vi "RestartImagingWNewParameters.vi"(8 "error IO":errorcluster, 11 "notifier out":refnum<notifier>) -> (0 "error out 2":errorcluster)   [LabVIEW 2015]
uses:
  NIDAQControls/StateGlobals.vi
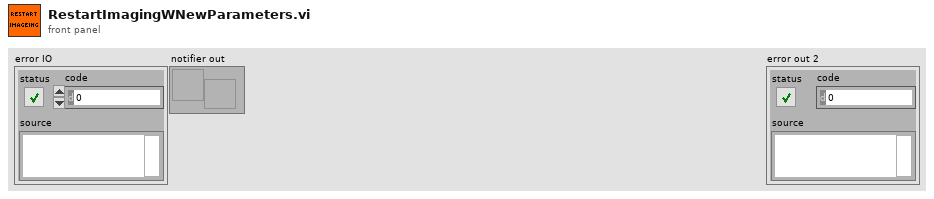
[diagram p1: front panel]
types:
  T1 = enum16{"Create", "Lossy Enqueue", "Enqueue", "Dequeue", "Destroy"}
  T2 = enum32{"Invalid", "Standard", "Closed", "Hidden", "Minimized", "Maximized"}
  T3 = cluster{"Start or New Parameters?":bool, "Laser Mode":string, "Piezo Mode":string, "Begin Or End Acquisition":string, "Acquisition Time":dbl}
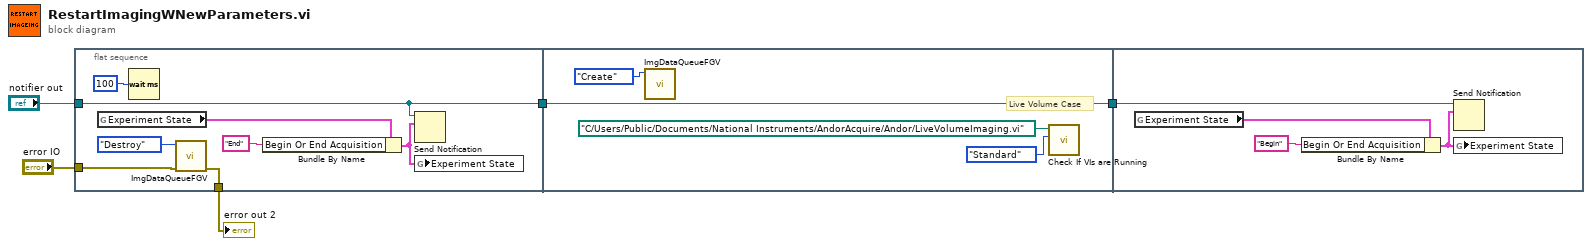
[diagram p0: block diagram]
diagram:
  n1 = flat-sequence {
    tunnel: "notifier out" -> [w6]
    tunnel: [w6] -> w5
    tunnel: "error IO" -> [w8]
    tunnel: [w7] -> w2
    tunnel: w5 -> [w17]
    tunnel: [w17] -> w4
    tunnel: w4 -> [w21]
    frame #0 {
      n2 = global read "StateGlobals.vi" "Experiment State"() -> (w13:T3)
      n3 = Wait (ms)(milliseconds to wait=u32 100) -> ()  [unwired: 1 out]
      n4 = call "ImgDataQueueFGV.vi"("error out"=w8, "Action"=T1."Destroy") -> ("error out 2"=w7:errorcluster)  [unwired: 7 in, 2 out]
      n5 = Bundle By Name(cluster=w13, "Begin Or End Acquisition"="End") -> (w11:T3)
      n6 = Send Notification(notification=w11, notifier=w6) -> ()  [unwired: 1 in, 2 out]
      n7 = global write "StateGlobals.vi" "Experiment State"(w11) -> ()
    }
    frame #1 {
      # "Live Volume Case"
      n8 = call "ImgDataQueueFGV.vi"("Action"=T1."Create") -> ()  [unwired: 8 in, 3 out]
      n9 = call "Check If VIs are Running.vi"("State"=T2."Standard", "Path"=path "C:/Users/Public/Documents/National Instruments/AndorAcquire/Andor/LiveVolumeImaging.vi") -> ()  [unwired: 9 in, 1 out]
    }
    frame #2 {
      n10 = global read "StateGlobals.vi" "Experiment State"() -> (w20:T3)
      n11 = Bundle By Name(cluster=w20, "Begin Or End Acquisition"="Begin") -> (w18:T3)
      n12 = Send Notification(notification=w18, notifier=w21) -> ()  [unwired: 1 in, 2 out]
      n13 = global write "StateGlobals.vi" "Experiment State"(w18) -> ()
    }
  }
  "error out 2" <- w2
